vi "PH_HamamatsuCamera.get ROI.vi"(0 "i ref in":refnum<vi>, 1 "Cam Handle in":i32, 4 "Cam Error in":errorcluster, 5 "error in (no error)":errorcluster) -> (14 "i ref out":refnum<vi>, 15 "Handle out":i32, 18 "Cam Error out":errorcluster, 19 "error out":errorcluster)   [LabVIEW 2014, in "PH_HamamatsuCamera.lvlib"]
doc: "This VI gets the ROI of the cam, and sets them to the GUI element and to own attributes."
uses:
  PH_HamamatsuCamera.lvlib
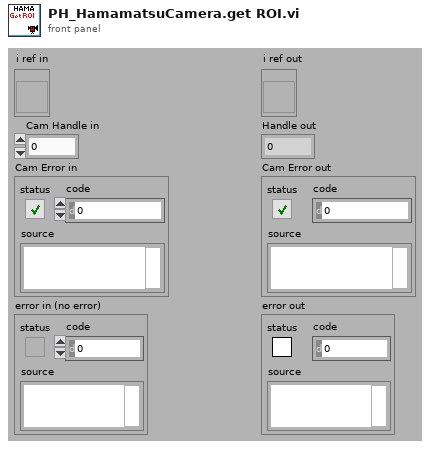
[diagram p1: front panel]
types:
  T1 = typedef "PH_HamamatsuCamera.lvlib/PH_HamamatsuCamera.i attribute.ctl" = cluster{"Gui Refs":cluster{"Camera Details":refnum<vi>, "ROI":refnum<vi>, "Set ROI to Maximum":refnum<vi>, "Trigger Parameters":refnum<vi>, "Brightness":refnum<vi>, "Shutter":refnum<vi>, "Gain":refnum<vi>, "Trigger Timeout":refnum<vi>, "Trigger Polarity":refnum<vi>, "Trigger Mode":refnum<vi>, "Parameters":refnum<vi>, "Set Cam Parameter":refnum<vi>, "Parameter to set":refnum<vi>, "Value to set":refnum<vi>}, "Cam":cluster{"Handle":i32, "Details":cluster{"Model":string, "Camera ID":string, "Firmware":string}, "Buffer Info":cluster{"height":u32, "width":u32, "datatype":u32}}, "H Offset":cluster{"Value":i32, "Minimum":i32, "Maximum":i32, "Increment":i32}, "V Offset":cluster{"Value":i32, "Minimum":i32, "Maximum":i32, "Increment":i32}, "H Width":cluster{"Value":i32, "Minimum":i32, "Maximum":i32, "Increment":i32}, "V Width":cluster{"Value":i32, "Minimum":i32, "Maximum":i32, "Increment":i32}, "Trigger Parameters":T2, "Trigger Timeout":u32, "Parameters":T3[], "Indicees Cam Parameters":cluster{"Brightness":i32, "Shutter":i32, "Gain":i32}, "Wanted Values":cluster{"Trigger Settings":T2[], "ROI":T4[], "Parameter":cluster{"Name":string, "Value":dbl}[]}}
  T2 = typedef "PH_HamamatsuCamera.lvlib/PH_HamamatsuCamera.Trigger Parameter.ctl" = cluster{"Mode":u32, "Polarity":u32, "Times":u32, "Delay":dbl}
  T3 = typedef "PH_HamamatsuCamera.lvlib/PH_HamamatsuCamera.Parameter Set.ctl" = cluster{"Parameter":string, "Value":dbl, "Writable":bool, "Range":cluster{"min":dbl, "max":dbl, "step":dbl}, "Default":dbl, "Value Names":cluster{"Name":string, "Value":dbl}[], "Text Values":bool}
  T4 = typedef "PH_HamamatsuCamera.lvlib/PH_HamamatsuCamera.ROI.ctl" = cluster{"Horizontal Offset":i32, "Vertical Offset":i32, "Horizontal Width":i32, "Vertical Width":i32}
  T5 = cluster{"Value":i32, "Minimum":i32, "Maximum":i32, "Increment":i32}
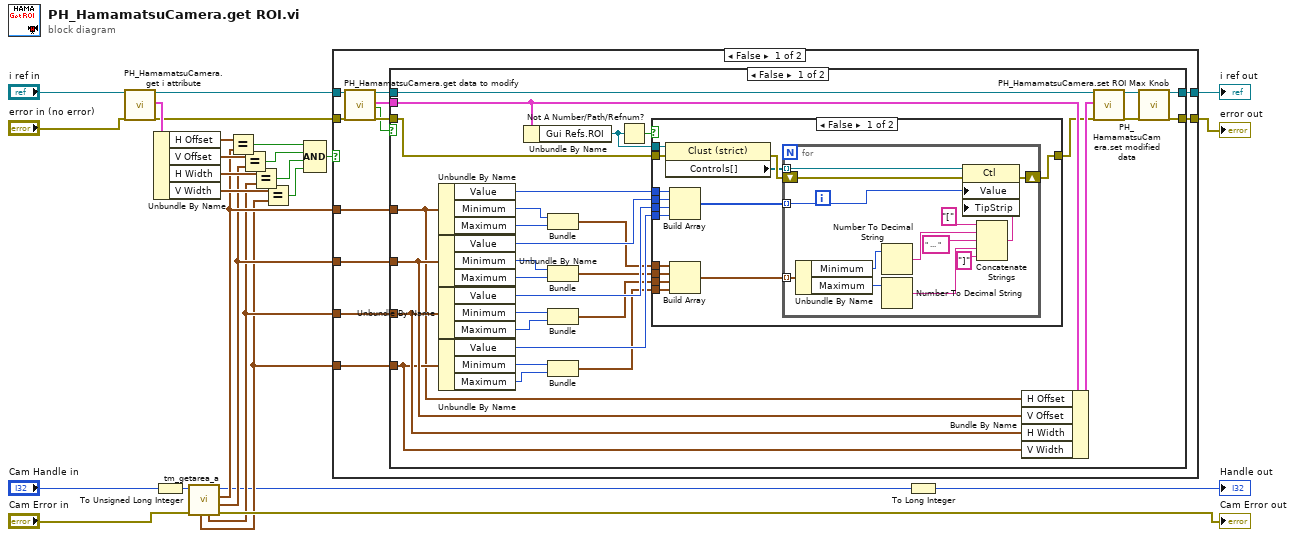
[diagram p0: block diagram]
diagram:
  n1 = call "PH_HamamatsuCamera.get i attribute.vi"("i ref in"="i ref in", "error in (no error)"="error in (no error)") -> ("i ref out"=w17:refnum<vi>, "i attribute"=w26:T1, "error out"=w15:errorcluster)  [unwired: 15 in]
  n2 = Unbundle By Name(w26) -> ("H Offset"=w21:T5, "V Offset"=w20:T5, "H Width"=w19:T5, "V Width"=w18:T5)
  n3 = To Unsigned Long Integer(number="Cam Handle in") -> (unsigned 32bit integer=w2:u32)
  n4 = call <userlib>:"tm_getarea_a.vi"("error in (no error)"="Cam Error in", "Handle in"=w2) -> ("error out"=→"Cam Error out":errorcluster, "V Offset"=w6:T5, "H Offset"=w7:T5, "Handle out"=w1:u32, "H Width"=w5:T5, "V Width"=w4:T5)  [unwired: 4 in]
  n5 = Equal?(x=w21, y=w7) -> (x = y?=w11:bool)
  n6 = Equal?(x=w20, y=w6) -> (x = y?=w10:bool)
  n7 = Equal?(x=w19, y=w5) -> (x = y?=w9:bool)
  n8 = Equal?(x=w18, y=w4) -> (x = y?=w8:bool)
  n9 = Compound Arithmetic op=AND(w11, w10, w9, w8) -> (w3:bool)
  n10 = case shown="False" w3 {
    tunnel: w15 -> [w38 w101]
    tunnel: [w36 w101] -> w22
    tunnel: w17 -> [w35 w102]
    tunnel: [w33 w102] -> w23
    tunnel: w7 -> [w31 _]
    tunnel: w6 -> [w30 _]
    tunnel: w5 -> [w29 _]
    tunnel: w4 -> [w28 _]
    frame False {
      n11 = call "PH_HamamatsuCamera.get data to modify.vi"("i ref in"=w35, "error in (no error)"=w38) -> ("i ref out"=w34:refnum<vi>, "i attribute"=w32:T1, "timed out"=w27:bool, "error out"=w37:errorcluster)  [unwired: 14 in]
      n12 = case shown="False" w27 {
        tunnel: w37 -> [w68 w99]
        tunnel: [w40 w99] -> w36
        tunnel: w34 -> [w67 w100]
        tunnel: [w41 w100] -> w33
        tunnel: w32 -> [w66 _]
        tunnel: w31 -> [w60 _]
        tunnel: w30 -> [w63 _]
        tunnel: w29 -> [w62 _]
        tunnel: w28 -> [w61 _]
        frame False {
          n13 = Unbundle By Name(w60) -> ("Value"=w59:i32, "Minimum"=w48:i32, "Maximum"=w49:i32)
          n14 = Unbundle By Name(w63) -> ("Value"=w58:i32, "Minimum"=w51:i32, "Maximum"=w50:i32)
          n15 = Unbundle By Name(w62) -> ("Value"=w57:i32, "Minimum"=w53:i32, "Maximum"=w52:i32)
          n16 = Unbundle By Name(w61) -> ("Value"=w56:i32, "Minimum"=w55:i32, "Maximum"=w54:i32)
          n17 = Unbundle By Name(w66) -> ("Gui Refs.ROI"=w65:refnum<vi>)
          n18 = Bundle("Minimum"=w48, "Maximum"=w49) -> (w44:cluster{"Minimum":i32, "Maximum":i32})  [unwired: 1 in]
          n19 = Bundle("Minimum"=w51, "Maximum"=w50) -> (w45:cluster{"Minimum":i32, "Maximum":i32})  [unwired: 1 in]
          n20 = Bundle("Minimum"=w53, "Maximum"=w52) -> (w46:cluster{"Minimum":i32, "Maximum":i32})  [unwired: 1 in]
          n21 = Bundle("Minimum"=w55, "Maximum"=w54) -> (w47:cluster{"Minimum":i32, "Maximum":i32})  [unwired: 1 in]
          n22 = Not A Number/Path/Refnum?(number/path/refnum=w65) -> (NaN/Path/Refnum?=w69:bool)
          n23 = case shown="False" w69 {
            tunnel: w65 -> [w84 _]
            tunnel: w68 -> [w83 w98]
            tunnel: [w81 w98] -> w43
            tunnel: w59 -> [w74 _]
            tunnel: w58 -> [w73 _]
            tunnel: w57 -> [w72 _]
            tunnel: w56 -> [w71 _]
            tunnel: w47 -> [w79 _]
            tunnel: w46 -> [w78 _]
            tunnel: w45 -> [w77 _]
            tunnel: w44 -> [w76 _]
            frame False {
              n24 = property class="Clust (strict)"(reference=w84, error in=w83) -> (error out=w82:errorcluster, "Controls[]"=w80:refnum<vi>[])  [unwired: 1 out]
              n25 = Build Array(w74, w73, w72, w71) -> (w70:i32[])
              n26 = Build Array(w76, w77, w78, w79) -> (w75:cluster{"Minimum":i32, "Maximum":i32}[])
              n27 = for {
                shift-right: [w95] -> w81
                shift-left: w82 -> [w97]
                tunnel: w80 -> [w96] mode=indexing
                tunnel: w75 -> [w93] mode=indexing
                tunnel: w70 -> [w94] mode=indexing
                n28 = Unbundle By Name(w93) -> ("Minimum"=w92:i32, "Maximum"=w91:i32)
                n29 = Number To Decimal String(number=w92) -> (decimal integer string=w89:string)  [unwired: 1 in]
                n30 = Number To Decimal String(number=w91) -> (decimal integer string=w88:string)  [unwired: 1 in]
                n31 = Concatenate Strings("[", w89, " ... " ("string"), w88, "]" ("string")) -> (w85:string)
                n32 = property class="Ctl"(reference=w96, error in=w97, "Value"=w94, "TipStrip"=w85) -> (error out=w95:errorcluster)  [unwired: 1 out]
              }
            }
            frame True {
            }
          }
          n33 = Bundle By Name(cluster=w66, "H Offset"=w60, "V Offset"=w63, "H Width"=w62, "V Width"=w61) -> (w64:T1)
          n34 = call "PH_HamamatsuCamera.set modified data.vi"("i ref in"=w67, "i attribute"=w64, "error in (no error)"=w43) -> ("i ref out"=w42:refnum<vi>, "error out"=w39:errorcluster)  [unwired: 15 in]
          n35 = call "PH_HamamatsuCamera.set ROI Max Knob.vi"("VI in"=w42, "error in (no error)"=w39) -> ("VI out"=w41:refnum<vi>, "error out"=w40:errorcluster)  [unwired: 16 in]
        }
        frame True {
        }
      }
    }
    frame True {
    }
  }
  "error out" <- w22
  "i ref out" <- w23
  n36 = To Long Integer(number=w1) -> (32bit integer=→"Handle out":i32)
